vi "Launch Connection Loop.vi"(8 "error in (no error)":errorcluster, 11 "TCP Client in":refnum<class "TCP Client.lvclass">) -> (0 "error out":errorcluster, 3 "TCP Client out":refnum<class "TCP Client.lvclass">)   [LabVIEW 2024, in "Stream-TCP.lvlib" / "TCP Client.lvclass"]
uses:
  TCP Client.lvclass
  C:/dev/lv20CE/relink/lv-stream/stream/Connection/Connection.lvclass
  lv-stream/stream/Connection/State.ctl
  TCP Client.lvclass/TCP Client.ctl
  lv-stream/stream/Connection/Connection.lvclass
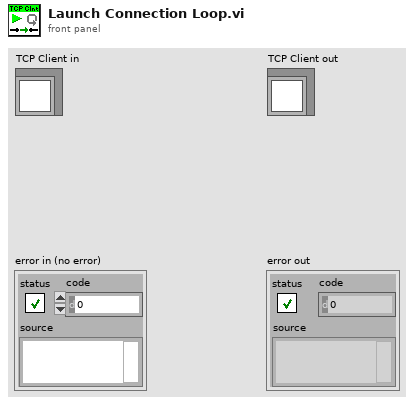
[diagram p1: front panel]
types:
  T1 = typedef "Stream.lvlib/Connection.lvclass/State.ctl" = enum16{"Closed", "Idle", "Connecting", "Connected", "Shutdown"}
  T2 = typedef "Stream-TCP.lvlib/TCP Client.lvclass/Ref Data.ctl" = cluster{"TCP Connection":refnum<k5>, "TCP Stream":refnum<class "TCP Stream.lvclass">, "Connection Loop":refnum<vi>, "Timeout ms":i32, "Server Connection":bool, "Open":bool}
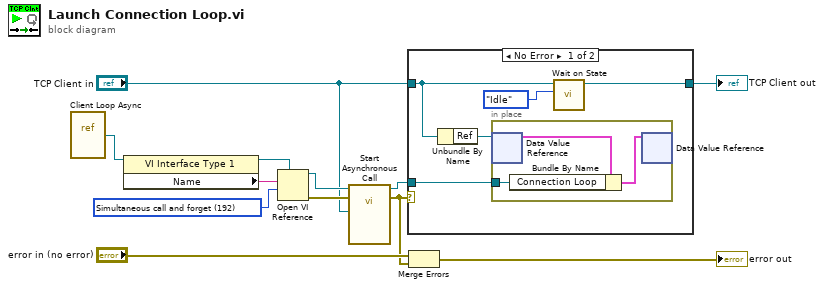
[diagram p0: block diagram]
diagram:
  w8 = 192 items=["Record modifications"=1, "Open templates for editing"=2, "Prompt user to save"=4, "Prepare for reentrant run"=8, "Prompt to find missing subVIs"=16, "Hide loading dialog box"=32, "Enable simultaneous calls"=64, "Prepare to call and forget"=128, "Simultaneous call and forget"=192, "Prepare to call and collect"=256, "Simultaneous call and collect"=320]
  n1 = vi-ref "Client Loop Async.vi"() -> (w6:refnum<vi>)
  n2 = property class="VI Interface Type 1"(reference=w6) -> (reference out=w9:refnum<vi>, "Name"=w7:string)  [unwired: 1 in, 1 out]
  n3 = Open VI Reference(type specifier VI Refnum (for type only)=w9, vi path=w7, options=w8) -> (vi reference=w11:refnum<vi>, error out=w10:errorcluster)  [unwired: 3 in]
  n4 = call-by-ref "Start Asynchronous Call"(reference=w11, error in=w10, "TCP Client in"="TCP Client in") -> (reference out=w3:refnum<vi>, error out=w4:errorcluster)  [unwired: 11 in]
  n5 = case shown="No Error" w4 {
    tunnel: w3 -> [w16 _]
    tunnel: "TCP Client in" -> [w15 w21]
    tunnel: [w14 w21] -> w1
    frame No Error {
      n6 = Unbundle By Name(w15) -> ("Ref"=w17:refnum<data-value>)
      n7 = in-place {
        in-place-border: w16 -> [w18]
        n8 = in-place-dvr #1(w17) -> (w20:T2)  [unwired: 1 out]
        n9 = Bundle By Name(cluster=w20, "Connection Loop"=w18) -> (w19:T2)
        n10 = in-place-dvr #1(w19) -> ()  [unwired: 2 out]
      }
      n11 = call "Wait on State.vi"("State"=State."Idle", "Connection in"=w15) -> ("Connection out"=w14:refnum<class "TCP Client.lvclass">)  [unwired: 7 in, 2 out]
    }
    frame Error {
    }
  }
  "TCP Client out" <- w1
  n12 = Merge Errors("error in (no error)", w4) -> (→"error out":errorcluster)
